vi "Test RS.vi"() -> ()   [LabVIEW 2014]
uses:
  Main-Stage-Based/(Global) Current handle and LaserPower_YCC.vi
panel:
  in  "T=growth\nF=back and forth":bool
  out "Numeric":dbl
  out "Axis":i32
  in  "T=extend\nF=contract":bool=TRUE
  in  "# of Step":dbl=5.0
  in  "Dwell time (ms)":dbl=500.0
  in  "Step (nm)":dbl=5.0
  in  "T=X\nF=Y":bool=TRUE
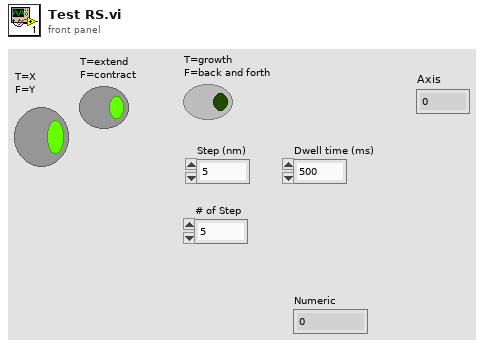
[diagram p1: front panel]
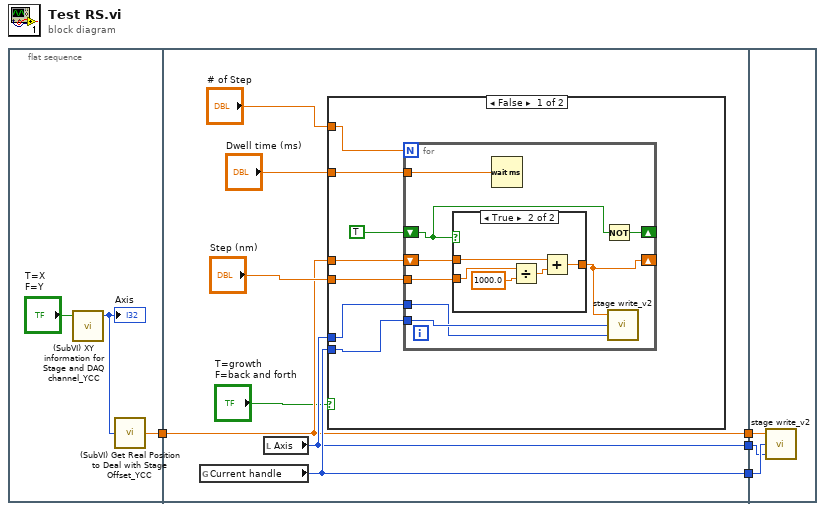
[diagram p0: block diagram]
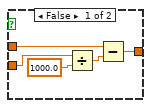
[diagram p2: hidden frame]
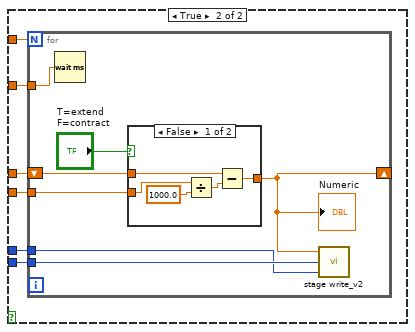
[diagram p3: hidden frame]
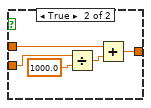
[diagram p4: hidden frame]
diagram:
  n1 = flat-sequence {
    tunnel: [w5] -> w4
    tunnel: w4 -> [w9]
    tunnel: [w11] -> w3
    tunnel: [w10] -> w2
    tunnel: [w9] -> w1
    tunnel: w3 -> [w65]
    tunnel: w2 -> [w64]
    tunnel: w1 -> [w63]
    frame #0 {
      n2 = call "(SubVI) XY information for Stage and DAQ channel_YCC.vi"("T=X\nF=Y"="T=X\nF=Y") -> ("Axis"=w6:i32)  [unwired: 3 in, 1 out]
      "Axis" <- w6
      n3 = call "(SubVI) Get Real Position to Deal with Stage Offset_YCC.vi"("Axis"=w6) -> ("Real Current Commanded position (um)"=w5:dbl)  [unwired: 3 in, 1 out]
    }
    frame #1 {
      n4 = global read "(Global) Current handle and LaserPower_YCC.vi" "Current handle"() -> (w11:i32)
      n5 = local read "Axis"() -> (w10:i32)
      n6 = case shown="False" "T=growth\nF=back and forth" {
        tunnel: "# of Step" -> [w16 w45]
        tunnel: "Step (nm)" -> [w20 w44]
        tunnel: "Dwell time (ms)" -> [w15 w43]
        tunnel: w11 -> [w18 w42]
        tunnel: w10 -> [w17 w41]
        tunnel: w9 -> [w21 w40]
        frame False {
          n7 = for {
            N: w16 -> [_]
            tunnel: w20 -> [w28]
            shift-right: [w27] -> _
            shift-left: TRUE -> [w26]
            tunnel: w18 -> [w25]
            tunnel: w17 -> [w24]
            tunnel: w15 -> [w23]
            shift-right: [w22] -> _
            shift-left: w21 -> [w29]
            n8 = case shown="True" w26 {
              tunnel: w29 -> [w34 w38]
              tunnel: w28 -> [w33 w37]
              tunnel: [w30 w35] -> w22
              frame False {
                n9 = Divide(x=w33, y=1000.0) -> (x/y=w31:dbl)
                n10 = Subtract(x=w34, y=w31) -> (x-y=w30:dbl)
              }
              frame True {
                n11 = Divide(x=w37, y=1000.0) -> (x/y=w36:dbl)
                n12 = Add(x=w38, y=w36) -> (x+y=w35:dbl)
              }
            }
            n13 = Wait (ms)(milliseconds to wait=w23) -> ()  [unwired: 1 out]
            n14 = Not(x=w26) -> (.not. x?=w27:bool)
            n15 = call "stage write_v2.vi"("axis"=w24, "Incoming Handle"=w25, "position"=w22) -> ()  [unwired: 2 in, 1 out]
          }
        }
        frame True {
          n16 = for {
            N: w45 -> [_]
            tunnel: w44 -> [w50]
            tunnel: w42 -> [w49]
            tunnel: w41 -> [w48]
            tunnel: w43 -> [w47]
            shift-right: [w46] -> _
            shift-left: w40 -> [w51]
            n17 = Wait (ms)(milliseconds to wait=w47) -> ()  [unwired: 1 out]
            n18 = case shown="False" "T=extend\nF=contract" {
              tunnel: w51 -> [w57 w61]
              tunnel: w50 -> [w56 w60]
              tunnel: [w53 w58] -> w46
              frame False {
                n19 = Divide(x=w56, y=1000.0) -> (x/y=w54:dbl)
                n20 = Subtract(x=w57, y=w54) -> (x-y=w53:dbl)
              }
              frame True {
                n21 = Divide(x=w60, y=1000.0) -> (x/y=w59:dbl)
                n22 = Add(x=w61, y=w59) -> (x+y=w58:dbl)
              }
            }
            "Numeric" <- w46
            n23 = call "stage write_v2.vi"("axis"=w48, "Incoming Handle"=w49, "position"=w46) -> ()  [unwired: 2 in, 1 out]
          }
        }
      }
    }
    frame #2 {
      n24 = call "stage write_v2.vi"("axis"=w64, "Incoming Handle"=w65, "position"=w63) -> ()  [unwired: 2 in, 1 out]
    }
  }
